vi "Measuring Complete - AndreTec.vi"() -> ()   [LabVIEW 2014]
doc: "André Romero - 2016\nandretec@ifsc.usp.br\nIFSC - USP"
uses:
  C:/Users/user/Documents/Andre/AutoLAB/Autolab SDK 1.11/EcoChemie.Autolab.Sdk.dll
  EcoChemie.Autolab.Sdk.dll
panel:
  out "Measured data 2":cluster{dbl[], dbl[]}(graph)
  out "Numeric":i32
  in  "Abort":bool
  in  "stop":bool
  in  "Y axis Signal":string(combo)
  in  "X axis Signal":string(combo)
  out "Measured data":cluster{"Y":dbl[], "Y":dbl[]}[](graph)
  out "X axis value":dbl
  out "Y axis value":dbl
  out "Measurement active":bool
  out "Blacklisted Commands detected":bool
  in  "Load Procedure":path=path "C:/Program Files/Metrohm Autolab/Autolab SDK 1.11/Standard Nova Procedures/Cyclic voltammetry.nox"
  out "Autolab Connected":bool
  in  "Embedded Exe File":path=path "C:/Program Files/Metrohm Autolab/Autolab SDK 1.11/Hardware Setup Files/Adk.x"
  in  "Hardware Setup File":path=path "C:/Program Files/Metrohm Autolab/Autolab SDK 1.11/Hardware Setup Files/PGSTAT204/HardwareSetup.xml"
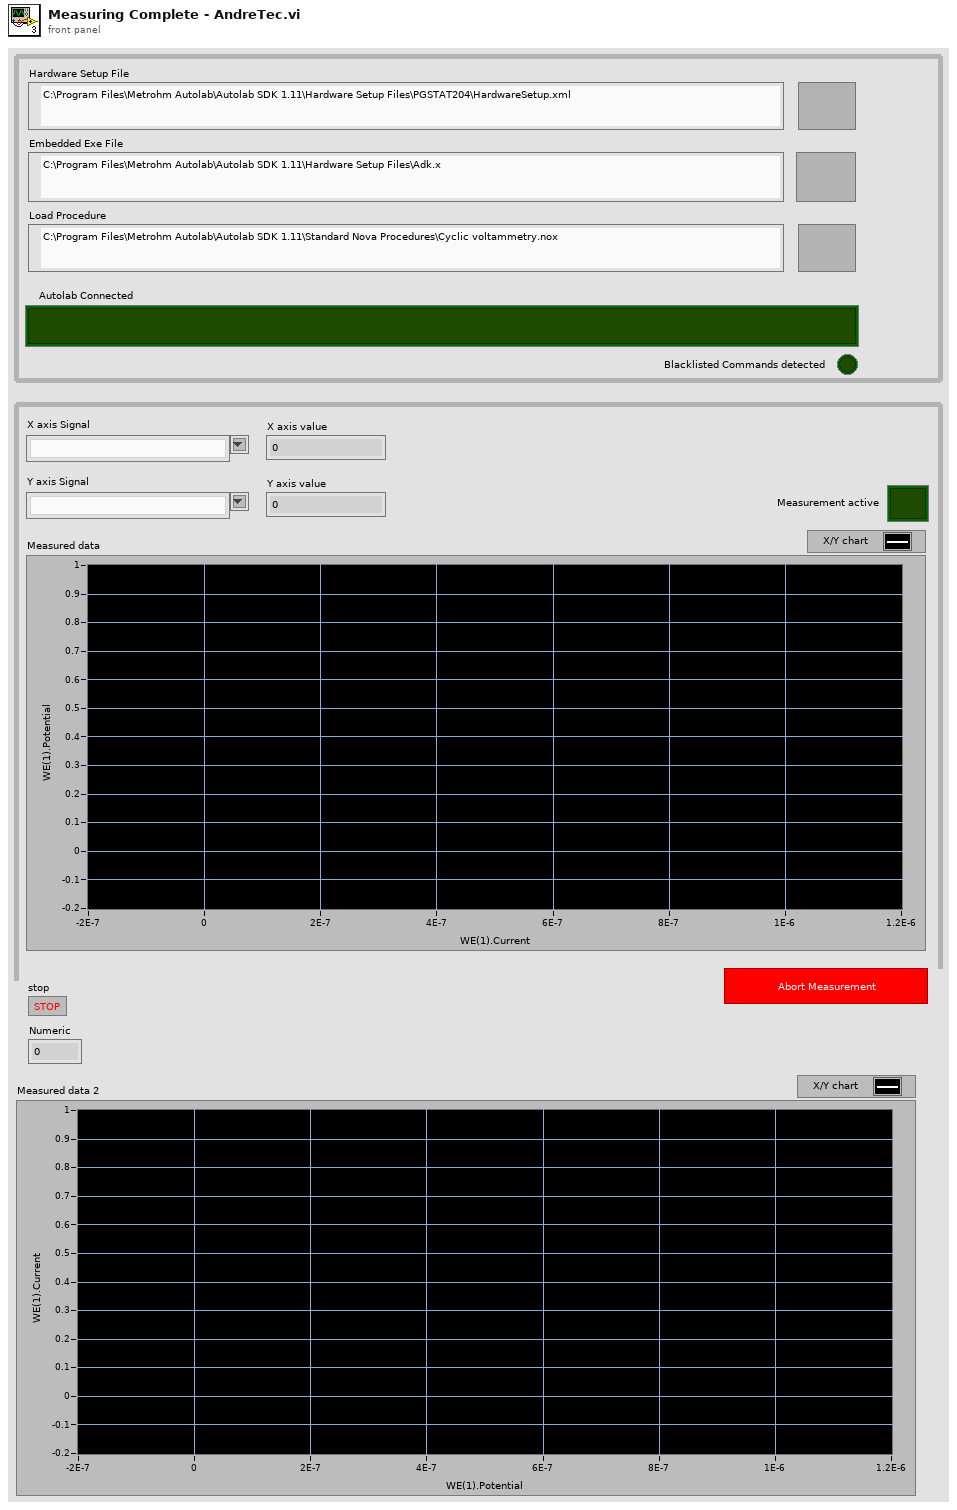
[diagram p1: front panel]
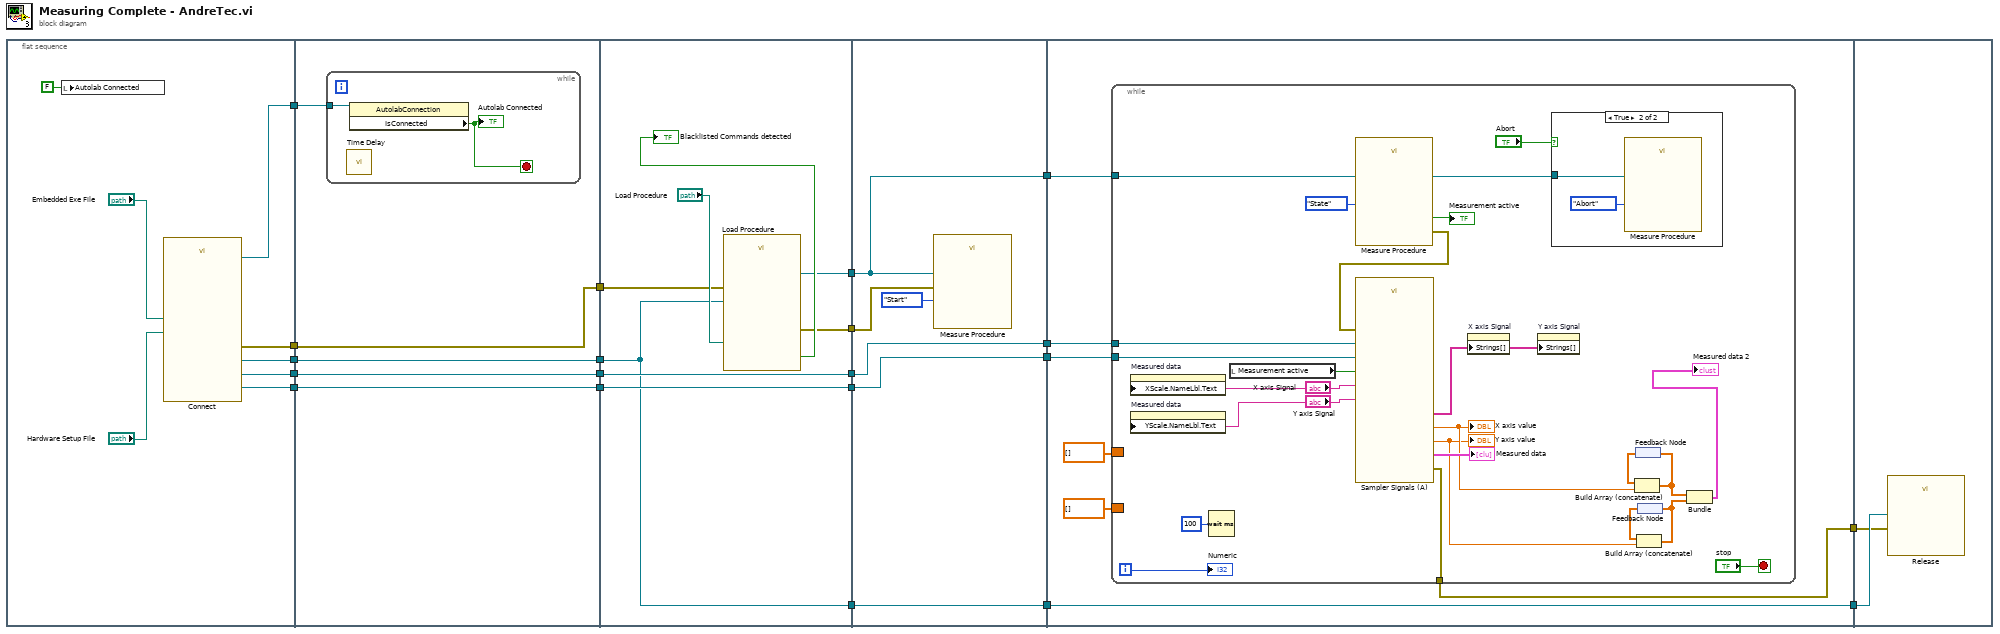
[diagram p0: block diagram]
diagram:
  n1 = flat-sequence {
    tunnel: [w26] -> w20
    tunnel: [w25] -> w18
    tunnel: [w24] -> w15
    tunnel: [w23] -> w13
    tunnel: [w22] -> w12
    tunnel: w20 -> [w33]
    tunnel: [w32] -> w19
    tunnel: w18 -> [w32]
    tunnel: w15 -> [w31]
    tunnel: [w31] -> w14
    tunnel: w13 -> [w30]
    tunnel: w12 -> [w29]
    tunnel: [w30] -> w10
    tunnel: [w29] -> w9
    tunnel: w19 -> [w36]
    tunnel: [w41] -> w17
    tunnel: [w40] -> w16
    tunnel: w14 -> [w39]
    tunnel: w10 -> [w38]
    tunnel: w9 -> [w37]
    tunnel: [w38] -> w8
    tunnel: [w37] -> w7
    tunnel: [w36] -> w3
    tunnel: w17 -> [w47]
    tunnel: w16 -> [w48]
    tunnel: [w47] -> w11
    tunnel: w8 -> [w46]
    tunnel: w7 -> [w45]
    tunnel: [w46] -> w6
    tunnel: [w45] -> w5
    tunnel: [w44] -> w4
    tunnel: w3 -> [w44]
    tunnel: w11 -> [w56]
    tunnel: w6 -> [w55]
    tunnel: w5 -> [w54]
    tunnel: w4 -> [w51]
    tunnel: [w51] -> w2
    tunnel: [w50] -> w1
    tunnel: w2 -> [w83]
    tunnel: w1 -> [w82]
    frame #0 {
      n2 = local write "Autolab Connected"(FALSE ("Autolab Connected")) -> ()
      n3 = call "Connect.vi"("Embedded Exe File"="Embedded Exe File", "Hardware Setup File"="Hardware Setup File") -> ("Sampler"=w23:refnum<k24>, "AutolabConnection"=w26:refnum<k24>, "instrument"=w25:refnum<k24>, "Ei"=w22:refnum<k24>, "error out"=w24:errorcluster)  [unwired: 1 in, 8 out]
    }
    frame #1 {
      n4 = while {
        tunnel: w33 -> [w34]
        stop <- w35 stop-if-true
        n5 = call "Time Delay"() -> ()  [unwired: 2 in, 10 out]
        n6 = property class="AutolabConnection"(reference=w34) -> ("IsConnected"=w35:bool)  [unwired: 1 in, 2 out]
        "Autolab Connected" <- w35
      }
    }
    frame #2 {
      n7 = call "Load Procedure.vi"("error in (no error)"=w39, "Procedure"="Load Procedure", "Instrument"=w36) -> ("error out"=w40:errorcluster, "Contains"=→"Blacklisted Commands detected":bool, "LoadProcedure"=w41:refnum<k24>)  [unwired: 6 out]
    }
    frame #3 {
      n8 = call "Measure Procedure.vi"("error in"=w48, "Request for procedure"=enum16{"State", "Save", "Abort", "Start"}."Start", "LoadProcedure"=w47) -> ()  [unwired: 1 in, 8 out]
    }
    frame #4 {
      n9 = while {
        tunnel: w56 -> [w68]
        tunnel: w55 -> [w71]
        tunnel: w54 -> [w70]
        border: dbl[] [] -> [_]
        border: dbl[] [] -> [_]
        tunnel: [w57] -> w50
        i -> [w65]
        stop <- "stop" stop-if-true
        n10 = property on="Measured data" class="XYGraph (strict)"("XScale.NameLbl.Text"="X axis Signal") -> ()  [unwired: 2 in, 2 out]
        n11 = property on="Measured data" class="XYGraph (strict)"("YScale.NameLbl.Text"="Y axis Signal") -> ()  [unwired: 2 in, 2 out]
        n12 = Wait (ms)(milliseconds to wait=u32 100) -> ()  [unwired: 1 out]
        n13 = local read "Measurement active"() -> (w74:bool)
        n14 = call "Measure Procedure.vi"("Request for procedure"=enum16{"State", "Save", "Abort", "Start"}."State", "LoadProcedure"=w68) -> ("error out"=w75:errorcluster, "IsMeasuring"=→"Measurement active":bool)  [unwired: 2 in, 6 out]
        n15 = call "Sampler Signals (A).vi"("IsMeasuring"=w74, "EI"=w70, "Sampler"=w71, "Signal X"="X axis Signal", "Signal Y"="Y axis Signal", "error in"=w75) -> ("X"=w63:dbl, "Y"=w61:dbl, "XY Graph"=→"Measured data":cluster{"Y":dbl[], "Y":dbl[]}[], "GetSignals"=w77:string[], "error out"=w57:errorcluster)  [unwired: 4 in, 1 out]
        "Y axis value" <- w61
        "X axis value" <- w63
        n16 = property on="X axis Signal" class="CmbBox"("Strings[]"=w77) -> ()  [unwired: 2 in, 2 out]
        n17 = property on="Y axis Signal" class="CmbBox"("Strings[]"=w77) -> ()  [unwired: 2 in, 2 out]
        n18 = case shown="True" "Abort" {
          tunnel: w68 -> [_ w80]
          frame False {
          }
          frame True {
            n19 = call "Measure Procedure.vi"("Request for procedure"=enum16{"State", "Save", "Abort", "Start"}."Abort", "LoadProcedure"=w80) -> ()  [unwired: 2 in, 8 out]
          }
        }
        n20 = feedback #1() -> (w64:dbl[])
        n21 = Build Array (concatenate)(w64, w63) -> (w60:dbl[])
        n22 = feedback-in #1(w60) -> ()
        n23 = feedback #2() -> (w62:dbl[])
        n24 = Build Array (concatenate)(w62, w61) -> (w59:dbl[])
        n25 = feedback-in #2(w59) -> ()
        n26 = Bundle(w60, w59) -> (→"Measured data 2":cluster{dbl[], dbl[]})  [unwired: 1 in]
        "Numeric" <- w65
      }
    }
    frame #5 {
      n27 = call "Release.vi"("error in (no error)"=w82, "Instrument"=w83) -> ()  [unwired: 1 in, 9 out]
    }
  }
